vi "Constructor.vi"(5 "TimeZoneInfoId":string, 7 "Time":timestamp, 8 "error in":errorcluster, 10 "Comment":string, 11 "Name":string) -> (0 "error out":errorcluster, 3 "UserComment out":refnum<class "UserComment.lvclass">)   [LabVIEW 2021, in "ProligentXMLGenerator.lvlib" / "UserComment.lvclass"]
uses:
  UserComment.lvclass
  UserComment.lvclass/UserComment.ctl
  Base/DateTime/DateTime.lvclass
  Base/NonEmptyString_255/NonEmptyString_255.lvclass
  Data.ctl
  Base/NonNullableString_TruncateAt_255/NonNullableString_TruncateAt_255.lvclass
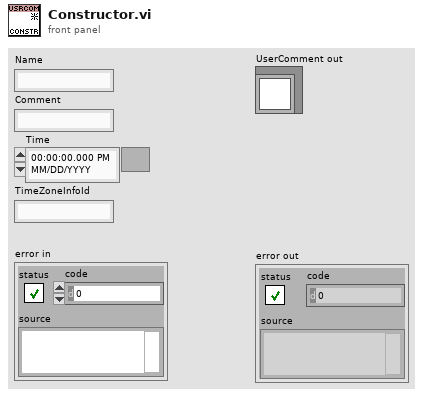
[diagram p1: front panel]
types:
  T1 = typedef "ProligentXMLGenerator.lvlib/UserComment.lvclass/Data.ctl" = cluster{"Name":string, "Comment":refnum<class "NonNullableString_TruncateAt_255.lvclass">, "User":refnum<class "NonEmptyString_255.lvclass">, "Time":refnum<class "DateTime.lvclass">}
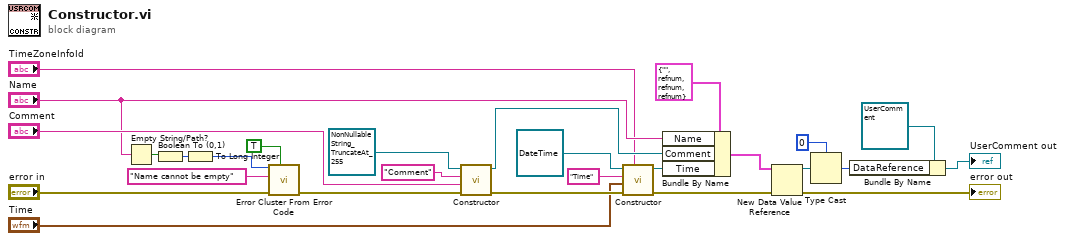
[diagram p0: block diagram]
diagram:
  n1 = Empty String/Path?(string/path="Name") -> (empty?=w12:bool)
  n2 = Boolean To (0,1)(Boolean=w12) -> (0, 1=w11:i16)
  n3 = To Long Integer(number=w11) -> (32bit integer=w10:i32)
  n4 = call <vilib>:"Error Cluster From Error Code.vi"("show call chain? (False)"=TRUE, "error in (no error)"="error in", "error message (\"\")"="Name cannot be empty" ("error message (\"\")"), "error code (0)"=w10) -> ("error out"=w8:errorcluster)  [unwired: 5 in]
  n5 = call-dynamic "Constructor.vi"("error in"=w8, "Value"="Comment", "Name"="Comment", "String in"=refnum<class "NonNullableString_TruncateAt_255.lvclass"> refnum ("NonNullableString_TruncateAt_255")) -> ("error out"=w16:errorcluster, "String out"=w18:refnum<class "NonNullableString_TruncateAt_255.lvclass">)  [unwired: 6 in]
  n6 = call-dynamic "Constructor.vi"("TimeZoneInfoId"="TimeZoneInfoId", "error in"=w16, "Value"="Time", "Name"="Time", "DateTime in"=refnum<class "DateTime.lvclass"> refnum ("DateTime.lvclass")) -> ("error out"=w6:errorcluster, "DateTime out"=w17:refnum<class "DateTime.lvclass">)  [unwired: 5 in]
  n7 = Bundle By Name(cluster=T1 {"Name"="", "Comment"=refnum, "User"=refnum, "Time"=refnum} ("Data"), "Name"="Name", "Comment"=w18, "Time"=w17) -> (w22:T1)
  n8 = New Data Value Reference(data value=w22, error in=w6) -> (data value reference=w21:refnum<data-value>, error out=→"error out":errorcluster)
  n9 = Type Cast(type=u64 0, x=w21) -> (*(type *) &x=w19:u64)
  n10 = Bundle By Name(cluster=refnum<class "UserComment.lvclass"> refnum ("ProligentResultProcessor:UserComment"), "DataReference"=w19) -> (→"UserComment out":refnum<class "UserComment.lvclass">)
